vi "PID turning.vi"(9 "Angle":dbl format="%.2f", 10 "GyroDevRef":T7={"DevStatus"={"status"=FALSE, "code"=0, "source"=""}, "Analog Channel"=enum."AI 1", "Gain (VoltsPerDegree/Second)"=0.0, "Gyro Type"=enum."Analog", "Handle"=0, "SPI Bus"=enum."Invalid", "Device Found"=FALSE, "Sample Rate"=1.0, "Calibrate On Open"=FALSE, "Offset"=0.0} {"Sample Rate" min=0.25 max=100.0 step=0.25}, 11 "RobotDriveDevRef":T1={"DevStatus"={"status"=FALSE, "code"=0, "source"=""}, "Motors[]"=[], "Square Inputs"=FALSE, "Max Output"=1.0}) -> (2 "GyroDevRef 2":T7={"DevStatus"={"status"=FALSE, "code"=0, "source"=""}, "Analog Channel"=enum."AI 1", "Gain (VoltsPerDegree/Second)"=0.0, "Gyro Type"=enum."Analog", "Handle"=0, "SPI Bus"=enum."Invalid", "Device Found"=FALSE, "Sample Rate"=1.0, "Calibrate On Open"=FALSE, "Offset"=0.0} {"Sample Rate" min=0.25 max=100.0 step=0.25}, 3 "RobotDriveDevRef 2":T1={"DevStatus"={"status"=FALSE, "code"=0, "source"=""}, "Motors[]"=[], "Square Inputs"=FALSE, "Max Output"=1.0})   [LabVIEW 2017]
uses:
  <vilib>/Rock Robotics/WPI/RobotDrive/WPI_RobotDriveDevRef.ctl
  <vilib>/Rock Robotics/WPI/MotorControl/WPI_MotorControlDeviceRef.ctl
  <vilib>/Rock Robotics/WPI/MotorControl/WPI_MotorControlType.ctl
  <vilib>/Rock Robotics/SystemInterfaces/DIO/FPGA_DIOPWMChannel.ctl
  <vilib>/Rock Robotics/WPI/PWM/WPI_PWMDeadband.ctl
  <vilib>/Rock Robotics/SystemInterfaces/DIO/FPGA_DIOChannel.ctl
  <vilib>/Rock Robotics/WPI/Gyro/WPI_GyroDevRef.ctl
  <vilib>/Rock Robotics/SystemInterfaces/AI/FPGA_AIChannel.ctl
  <vilib>/Rock Robotics/SystemInterfaces/spilib/spi_bus.ctl
  Robot Global Data.vi
  <vilib>/addons/control/pid/pid.llb/PID (DBL).vi
  <vilib>/addons/control/pid/NI_PID_pid.lvlib
panel:
  # "Analog"
  # "XRS"
  # "Analog"
  # "XRS"
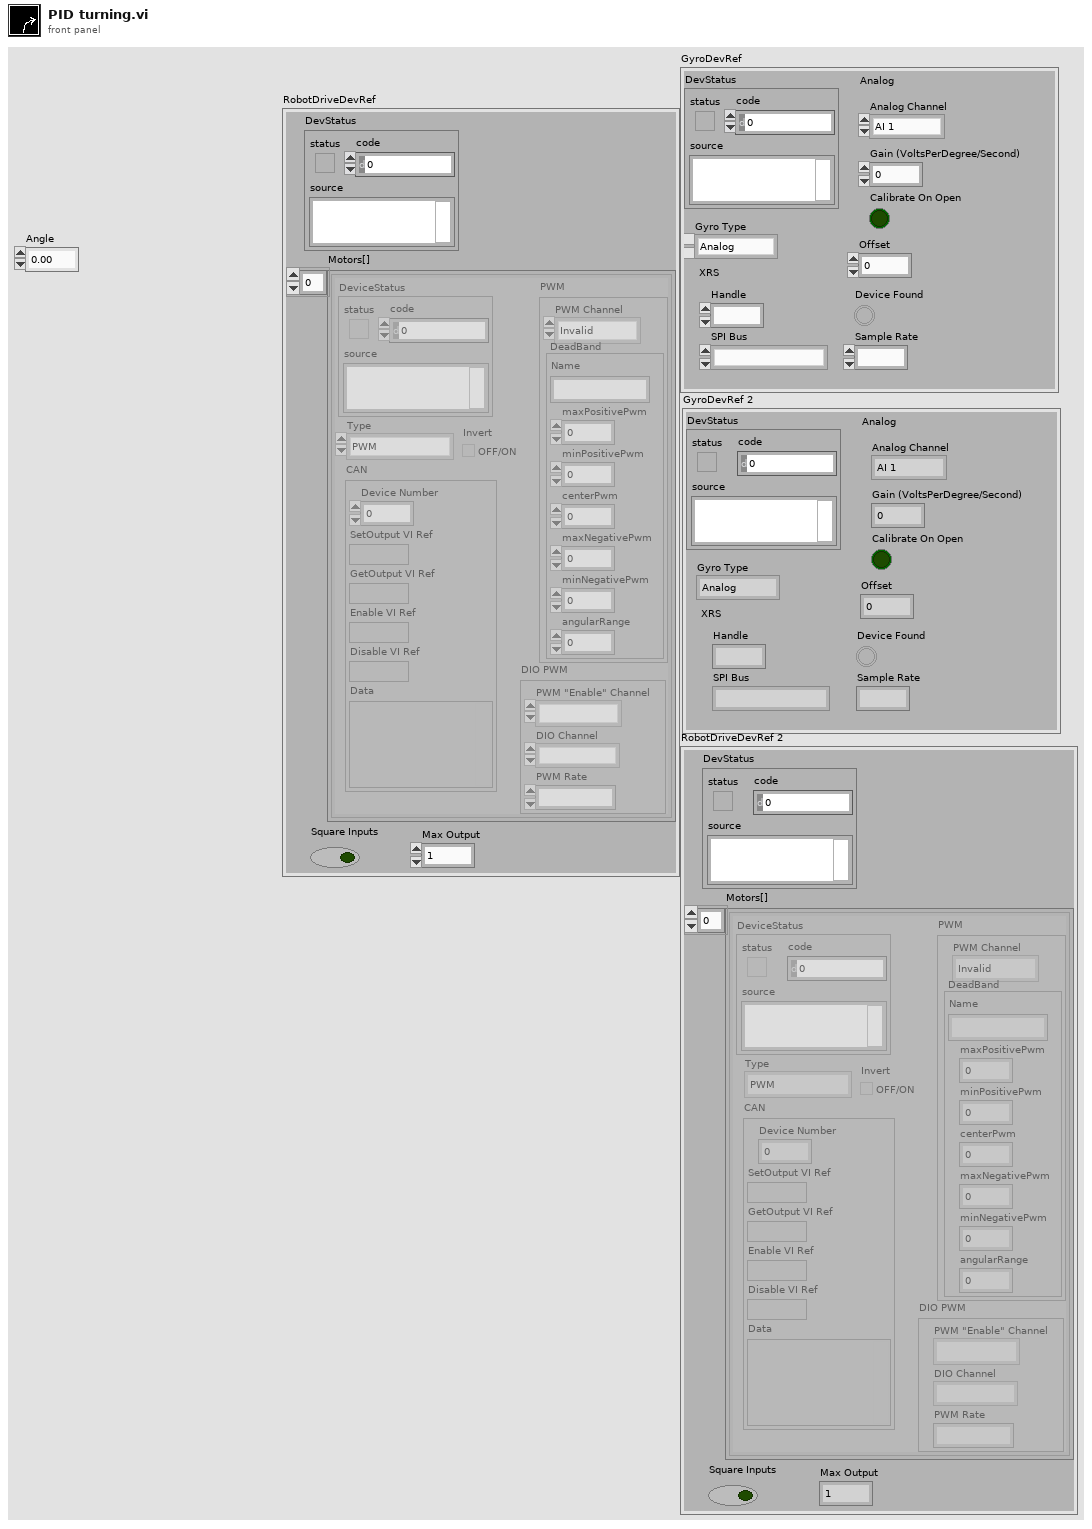
[diagram p1: front panel]
types:
  T1 = typedef "WPI_RobotDriveDevRef.ctl" = cluster{"DevStatus":errorcluster, "Motors[]":T2[], "Square Inputs":bool, "Max Output":dbl}
  T2 = typedef "WPI_MotorControlDeviceRef.ctl" = cluster{"DeviceStatus":errorcluster, "Type":T3, "PWM":cluster{"PWM Channel":T4, "DeadBand":T5}, "CAN":cluster{"Device Number":u8, "SetOutput VI Ref":variant, "GetOutput VI Ref":variant, "Enable VI Ref":variant, "Disable VI Ref":variant, "Data":variant}, "Invert":bool, "DIO PWM":cluster{"PWM \"Enable\" Channel":T4, "DIOChannel":T6, "PWM Rate":dbl}}
  T3 = typedef "WPI_MotorControlType.ctl" = enum16{"PWM", "CAN", "DIO PWM"}
  T4 = typedef "FPGA_DIOPWMChannel.ctl" = enum8{"PWM 0", "PWM 1", "PWM 2", "PWM 3", "PWM 4", "PWM 5", "PWM 6", "PWM 7", "PWM 8", "PWM 9", "PWM MXP 0", "PWM MXP 1", "PWM MXP 2", "PWM MXP 3", "PWM MXP 4", "PWM MXP 5", "PWM MXP 6", "PWM MXP 7", "PWM MXP 8", "PWM MXP 9", "Invalid"}
  T5 = typedef "WPI_PWMDeadband.ctl" = cluster{"Name":string, "maxPositivePwm":i32, "minPositivePwm":i32, "centerPwm":i32, "maxNegativePwm":i32, "minNegativePwm":i32, "angularRange":u16}
  T6 = typedef "FPGA_DIOChannel.ctl" = enum8{"DIO 0", "DIO 1", "DIO 2", "DIO 3", "DIO 4", "DIO 5", "DIO 6", "DIO 7", "DIO 8", "DIO 9", "DIO MXP 0", "DIO MXP 1", "DIO MXP 2", "DIO MXP 3", "DIO MXP 4", "DIO MXP 5", "DIO MXP 6", "DIO MXP 7", "DIO MXP 8", "DIO MXP 9", "DIO MXP 10", "DIO MXP 11", "DIO MXP 12", "DIO MXP 13", "DIO MXP 14", "DIO MXP 15", "SPI Port CS1", "SPI Port CS2", "SPI Port CS3", "SPI Port MISO", "SPI Port MOSI", "Invalid"}
  T7 = typedef "WPI_GyroDevRef.ctl" = cluster{"DevStatus":errorcluster, "Analog Channel":T8, "Gain (VoltsPerDegree/Second)":dbl, "Gyro Type":enum16{"Analog", "XRS450"}, "Handle":i32, "SPI Bus":T9, "Device Found":bool, "Sample Rate":dbl, "Calibrate On Open":bool, "Offset":dbl}
  T8 = typedef "FPGA_AIChannel.ctl" = enum8{"AI 0", "AI 1", "AI 2", "AI 3", "AI MXP 0", "AI MXP 1", "AI MXP 2", "AI MXP 3", "Invalid"}
  T9 = typedef "spi_bus.ctl" = enum16{"SPI On-Board, CS0", "SPI On-Board, CS1", "SPI On-Board, CS2", "SPI On-Board, CS3", "SPI MXP", "Invalid"}
  T10 = cluster{"proportional gain (Kc)":dbl, "integral time (Ti, min)":dbl, "derivative time (Td, min)":dbl}
  T11 = cluster{"Motor Values[0]":dbl, "Motor Values[1]":dbl, "Motor Values[2]":dbl, "Motor Values[3]":dbl, "Motor Values[4]":dbl, "Motor Values[5]":dbl, "Motor Values[6]":dbl, "Motor Values[7]":dbl, "Motor Values[8]":dbl}
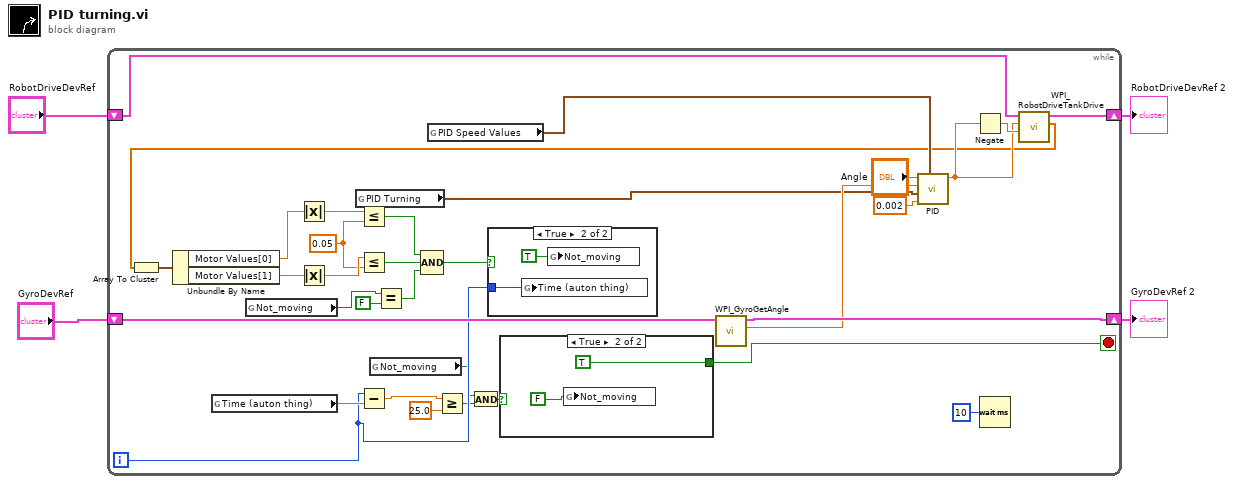
[diagram p0: block diagram]
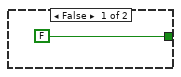
[diagram p2: hidden frame]
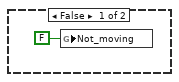
[diagram p3: hidden frame]
diagram:
  n1 = while {
    shift-right: [w36] -> w2
    shift-left: "GyroDevRef" -> [w37]
    shift-right: [w34] -> w1
    shift-left: "RobotDriveDevRef" -> [w35]
    i -> [w25]
    stop <- w19 stop-if-true
    w12 = 0.05 ("y")
    n2 = global read "Robot Global Data.vi" "Time (auton thing)"() -> (w26:dbl)
    n3 = global read "Robot Global Data.vi" "Not_moving"() -> (w11:bool)
    n4 = global read "Robot Global Data.vi" "PID Turning"() -> (w29:T10)
    n5 = Subtract(x=w25, y=w26) -> (x-y=w24:dbl)
    n6 = global read "Robot Global Data.vi" "Not_moving"() -> (w21:bool)
    n7 = Equal?(x=w11, y=FALSE) -> (x = y?=w7:bool)
    n8 = global read "Robot Global Data.vi" "PID Speed Values"() -> (w27:cluster{"Output High":dbl, "Output Low":dbl})
    n9 = Greater Or Equal?(x=w24, y=25.0) -> (x >= y?=w22:bool)
    n10 = And(x=w21, y=w22) -> (x .and. y?=w20:bool)
    n11 = case shown="True" w20 {
      tunnel: [FALSE TRUE] -> w19
      frame False {
      }
      frame True {
        n12 = global write "Robot Global Data.vi" "Not_moving"(FALSE ("Not_moving")) -> ()
      }
    }
    n13 = call <vilib>:"WPI_GyroGetAngle.vi"("GyroDevRef"=w37) -> ("Angle"=w33:dbl, "GyroDevRef"=w36:T7)  [unwired: 6 in, 3 out]
    n14 = call-poly <vilib>:"PID.vi"("output range"=w27, "dt (s)"=0.002, "PID gains"=w29, "process variable"=w33, "setpoint"="Angle") -> ("output"=w30:dbl)  [unwired: 5 in, 1 out]
    n15 = Negate(x=w30) -> (-x=w31:dbl)
    n16 = Wait (ms)(milliseconds to wait=u32 10) -> ()  [unwired: 1 out]
    n17 = call <vilib>:"WPI_RobotDriveTankDrive.vi"("Right axis value"=w31, "Left axis value"=w30, "RobotDriveDevRef"=w35) -> ("Motor Values"=w18:dbl[], "RobotDriveDevRef"=w34:T1)  [unwired: 6 in, 1 out]
    n18 = Array To Cluster(array=w18) -> (cluster=w17:T11)
    n19 = Unbundle By Name(w17) -> ("Motor Values[0]"=w16:dbl, "Motor Values[1]"=w15:dbl)
    n20 = Absolute Value(x=w16) -> (abs(x)=w14:dbl)
    n21 = Absolute Value(x=w15) -> (abs(x)=w13:dbl)
    n22 = Less Or Equal?(x=w14, y=w12) -> (x <= y?=w9:bool)
    n23 = Less Or Equal?(x=w13, y=w12) -> (x <= y?=w8:bool)
    n24 = Compound Arithmetic op=AND(w9, w8, w7) -> (w6:bool)
    n25 = case shown="True" w6 {
      tunnel: w25 -> [_ w43]
      frame False {
        n26 = global write "Robot Global Data.vi" "Not_moving"(FALSE ("Not_moving")) -> ()
      }
      frame True {
        n27 = global write "Robot Global Data.vi" "Time (auton thing)"(w43) -> ()
        n28 = global write "Robot Global Data.vi" "Not_moving"(TRUE ("Not_moving")) -> ()
      }
    }
  }
  "GyroDevRef 2" <- w2
  "RobotDriveDevRef 2" <- w1
